vi "LabVIEWSample.vi"(9 "Low Limit":dbl, 10 "High Limit":dbl, 11 "Nr Measure":i32) -> (3 "?":T1, 5 "Waveform Chart":T1(graph))   [LabVIEW 2013]
uses:
  <vilib>/Analysis/baseanly.llb/Mean (DBL).vi
  <vilib>/Utility/file.llb/Write To Spreadsheet File (DBL).vi
  <vilib>/Analysis/NI_AALBase.lvlib
panel:
  out "?":cluster{string, dbl, "mean":dbl, string, dbl}
  out "output cluster 3":cluster{string, bool, string, bool}
  out "Tem":dbl[][](array[numeric])
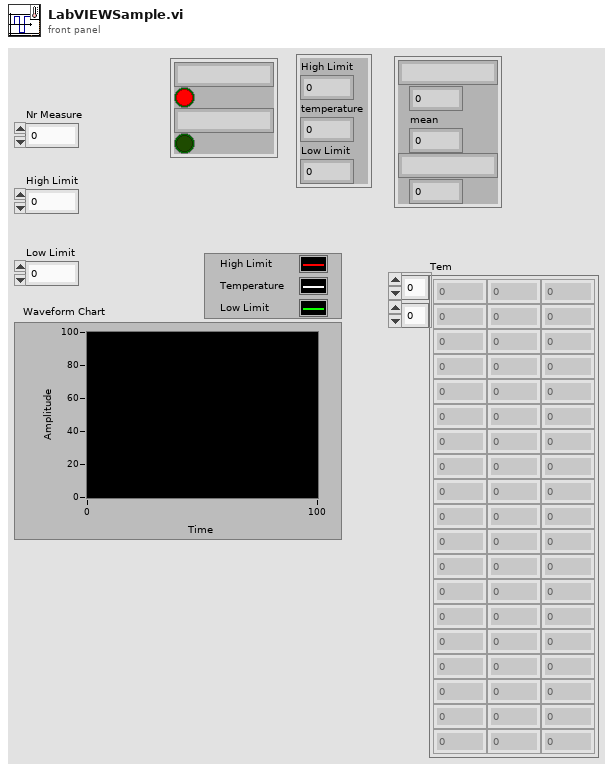
[diagram p1: front panel]
types:
  T1 = cluster{"High Limit":dbl, "temperature":dbl, "Low Limit":dbl}
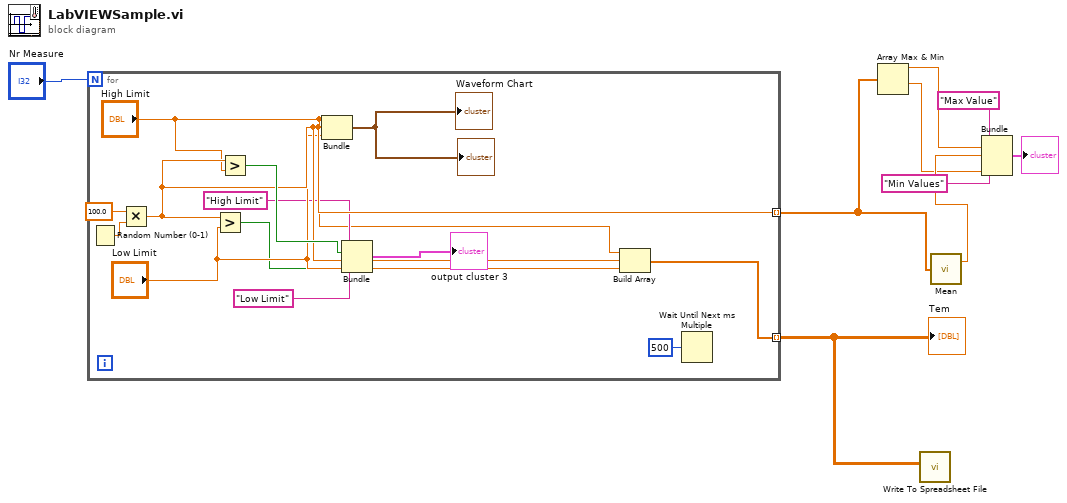
[diagram p0: block diagram]
diagram:
  n1 = for {
    N: "Nr Measure" -> [_]
    tunnel: [w17] -> w6 mode=indexing
    tunnel: [w15] -> w5 mode=indexing
    n2 = Random Number (0-1)() -> (number: 0 to 1=w20:dbl)
    n3 = Multiply(x=100.0, y=w20) -> (x*y=w17:dbl)
    n4 = Greater?(x=w17, y="Low Limit") -> (0:w13:bool)
    n5 = Greater?(x=w17, y="High Limit") -> (0:w22:bool)
    n6 = Bundle("High Limit"="High Limit", w17, "Low Limit"="Low Limit") -> (→"?" →"Waveform Chart":cluster{"High Limit":dbl, dbl, "Low Limit":dbl})  [unwired: 1 in]
    n7 = Bundle("High Limit", w22, "Low Limit", w13) -> (→"output cluster 3":cluster{string, bool, string, bool})  [unwired: 1 in]
    n8 = Build Array("High Limit", w17, "Low Limit") -> (w15:dbl[])
    n9 = Wait Until Next ms Multiple(millisecond multiple=u32 500) -> ()  [unwired: 1 out]
  }
  "Tem" <- w5
  n10 = Array Max & Min(array=w6) -> (max value=w8:dbl, min value=w3:dbl)  [unwired: 2 out]
  n11 = call-poly <vilib>:"Write To Spreadsheet File.vi"("2D data"=w5) -> ()  [unwired: 7 in, 1 out]
  n12 = call-poly <vilib>:"Mean.vi"("X"=w6) -> ("mean"=w7:dbl)  [unwired: 1 out]
  n13 = Bundle("Max Value", w8, "mean"=w7, "Min Values", w3) -> (→"?":cluster{string, dbl, "mean":dbl, string, dbl})  [unwired: 1 in]
